vi "init.vi"(8 "error in (no error)":errorcluster, 9 "height":dbl, 10 "width":dbl, 11 "Rectangle in":refnum<class "Rectangle.lvclass">) -> (0 "error out":errorcluster, 3 "Rectangle out":refnum<class "Rectangle.lvclass">)   [LabVIEW 2024, in "Rectangle.lvclass"]
uses:
  Rectangle.lvclass
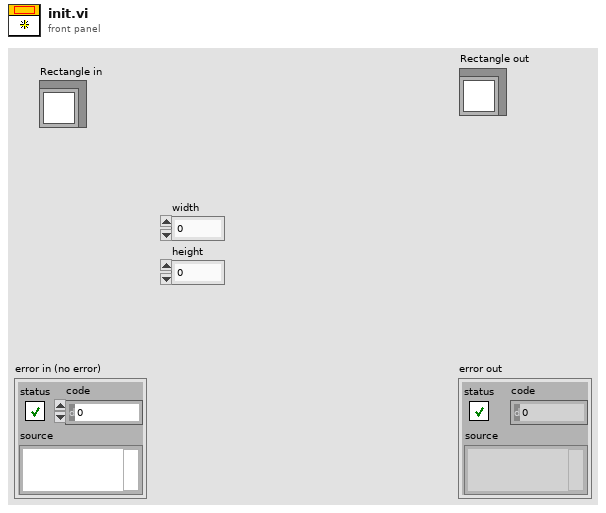
[diagram p1: front panel]
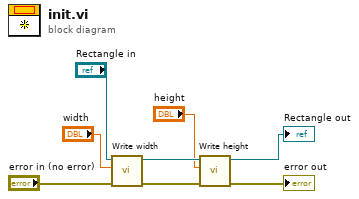
[diagram p0: block diagram]
diagram:
  n1 = call-dynamic "Write width.vi"("error in (no error)"="error in (no error)", "width"="width", "Rectangle in"="Rectangle in") -> ("error out"=w2:errorcluster, "Rectangle out"=w7:refnum<class "Rectangle.lvclass">)  [unwired: 7 in]
  n2 = call-dynamic "Write height.vi"("error in (no error)"=w2, "height"="height", "Rectangle in"=w7) -> ("error out"=→"error out":errorcluster, "Rectangle out"=→"Rectangle out":refnum<class "Rectangle.lvclass">)  [unwired: 7 in]
